vi "Configure Reference Waveform.vi"   [LabVIEW 2023, in "Keysight-DSQx3014T.lvlib"]
doc: "Configures reference waveform."
uses:
  Keysight-DSQx3014T.lvlib
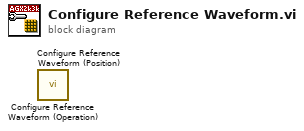
[diagram p0: block diagram]
diagram:
  n1 = call "Configure Reference Waveform (Operation).vi"() -> ()  [unwired: 10 in, 2 out]
  n2 = call "Configure Reference Waveform (Position).vi"() -> ()  [unwired: 10 in, 2 out]
